vi "even&odd1.vi"() -> ()   [LabVIEW 2020]
panel:
  out "String 3":string
  in  "negative":string
  in  "positive":string
  out "even":bool
  out "s? t:f":string
  in  "String":string
  in  "Numeric":dbl
  in  "String 2":string
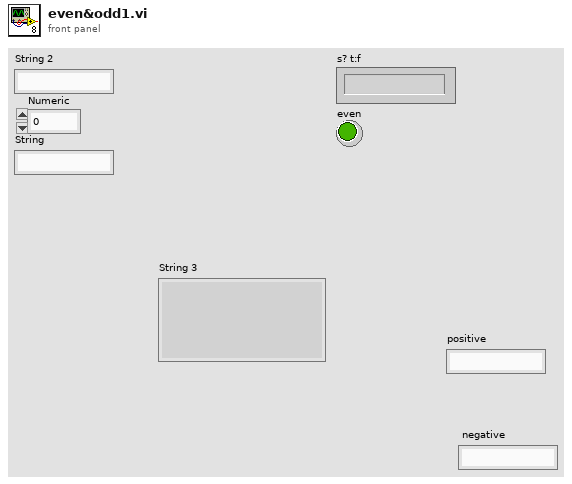
[diagram p1: front panel]
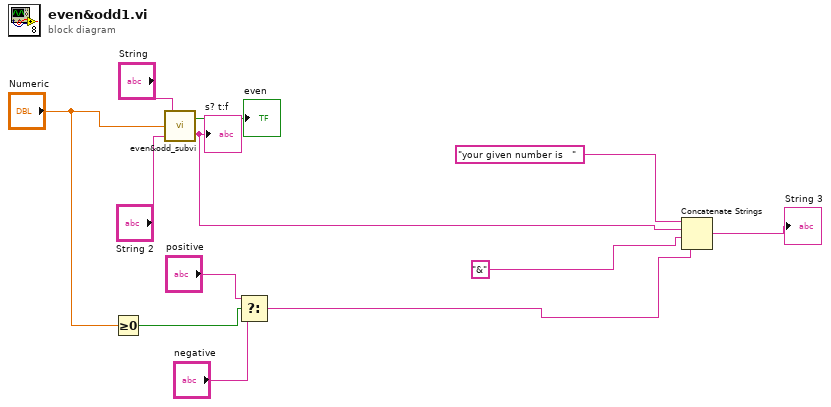
[diagram p0: block diagram]
diagram:
  n1 = Greater Or Equal To 0?(x="Numeric") -> (x >= 0?=w8:bool)
  n2 = call "even&odd_subvi.vi"("String 2"="String 2", "Numeric"="Numeric", "String"="String") -> ("s? t:f"=w4:string, "even"=→"even":bool)
  "s? t:f" <- w4
  n3 = Select(t="positive", s=w8, f="negative") -> (s? t:f=w2:string)
  n4 = Concatenate Strings("your given number is   " ("String 3"), w4, "&" ("positive"), w2) -> (→"String 3":string)
